vi "LinxPwmSetDutyCycle.vi"(8 "Error In":errorcluster, 9 "Duty Cycles":dbl[](array[numeric]), 10 "PWM Channels":u8[](array[numeric]), 11 "LINX Resource":T1) -> (0 "Error Out":errorcluster, 3 "LINX Resource":T1)   [LabVIEW 2020, in "LMH-LINX.lvlib" / "Local IO.lvlib"]
uses:
  Local IO.lvlib
  Type Defs/LINX Ref.ctl
  Type Defs/Platform.ctl
  Type Defs/Interface.ctl
  Device/Type Defs/LINX Device Config.ctl
  Device/Type Defs/TCP Config.ctl
  Device/Type Defs/Channels.ctl
  <vilib>/MakerHub/LINX/Resources/liblinxdevice.dll
  LMH-LINX.lvlib
  Device/Device.lvlib
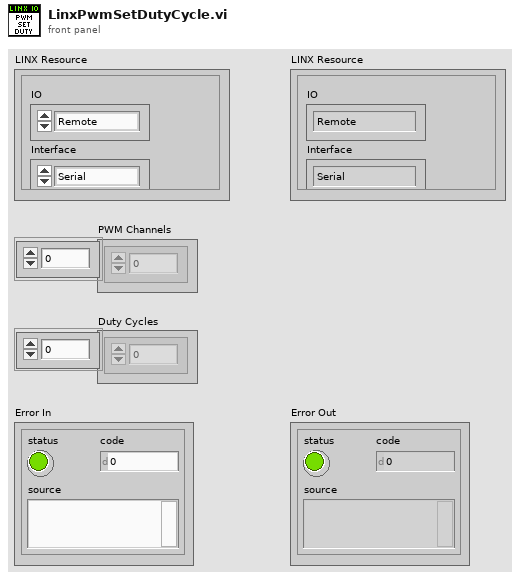
[diagram p1: front panel]
types:
  T1 = typedef "LMH-LINX.lvlib/LINX Ref.ctl" = cluster{"IO":T2, "Interface":T3, "LINX Device Config":T4}
  T2 = typedef "LMH-LINX.lvlib/Platform.ctl" = enum16{"Remote", "Local"}
  T3 = typedef "LMH-LINX.lvlib/Interface.ctl" = enum16{"Serial", "TCP"}
  T4 = typedef "LMH-LINX.lvlib/Device.lvlib/LINX Device Config.ctl" = cluster{"Interface":T3, "COM Port":refnum<visa-resource-name>, "TCP Configuration":T5, "Device Family":u8, "Device ID":u8, "Device Name":string, "TCP Ref":refnum<k5>, "Channels":T6}
  T5 = typedef "LMH-LINX.lvlib/Device.lvlib/TCP Config.ctl" = cluster{"IP Address":string, "Port":u16}
  T6 = typedef "LMH-LINX.lvlib/Channels.ctl" = cluster{"DI":u8[], "DO":u8[], "AI":u8[], "AO":u8[], "PWM":u8[], "QE":u8[], "UART":u8[], "I2C 2":u8[], "SPI":u8[], "CAN":u8[], "Servo":u8[], "AI Ref (V)":dbl, "AI Resolution (Bits)":u8, "AO Ref (V)":dbl, "AO Resolution (Bits)":u8}
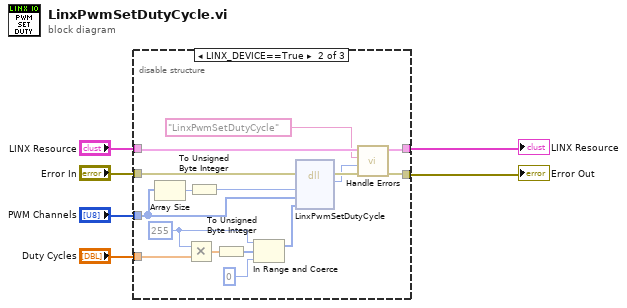
[diagram p0: block diagram]
diagram:
  n1 = disable-structure shown="LINX_DEVICE==True" {
    disable-tunnel: "LINX Resource" -> [w8 w23 w26]
    disable-tunnel: "Error In" -> [w7 w24 w25]
    disable-tunnel: [w7 w21 w25] -> w4
    disable-tunnel: [w8 w22 w26] -> w3
    disable-tunnel: "PWM Channels" -> [_ w15 _]
    disable-tunnel: "Duty Cycles" -> [_ w10 _]
    frame condition #0 (active) {
    }
    frame condition #1 {
      w14 = u8 255
      n2 = Array Size(array=w15) -> (size(s)=w16:i32)
      n3 = Multiply(x=w14, y=w10) -> (x*y=w13:dbl[])
      n4 = To Unsigned Byte Integer(number=w16) -> (unsigned 8bit integer=w17:u8)
      n5 = To Unsigned Byte Integer(number=w13) -> (unsigned 8bit integer=w12:u8[])
      n6 = In Range and Coerce(upper limit=w14, x=w12, lower limit=u8 0) -> (coerced(x)=w9:u8[])  [unwired: 1 out]
      n7 = dll-call lib="C:/Program Files (x86)/National Instruments/LabVIEW 2020/vi.lib/MakerHub/LINX/Resources/liblinxdevice.*" fn="LinxPwmSetDutyCycle"(error in=w24, "numChans"=w17, "channels"=w15, "values"=w9) -> (error out=w20:errorcluster, "LinxStatus"=w19:i32)  [unwired: 5 in, 1 out]
      n8 = call <vilib>:"Handle Errors.vi"("Error In"=w20, "LinxStatus"=w19, "Function Name"="LinxPwmSetDutyCycle", "LINX Resource"=w23) -> ("Error Out"=w21:errorcluster, "LINX Resource"=w22:T1)  [unwired: 6 in]
    }
    frame condition #2 {
    }
  }
  "Error Out" <- w4
  "LINX Resource" <- w3
